vi "Write Listener Port.vi"(8 "error in (no error)":errorcluster, 10 "Listener Port":u16=6341, 11 "Server Config in":refnum<class "Server Config.lvclass">) -> (0 "error out":errorcluster, 3 "Server Config out":refnum<class "Server Config.lvclass">)   [LabVIEW 2026, in "Server Controller.lvlib" / "Server Config.lvclass"]
uses:
  Server Config.lvclass
  Server Config.lvclass/Server Config.ctl
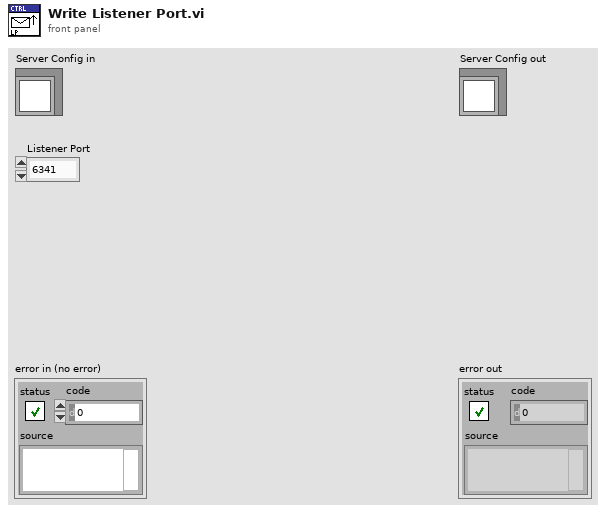
[diagram p1: front panel]
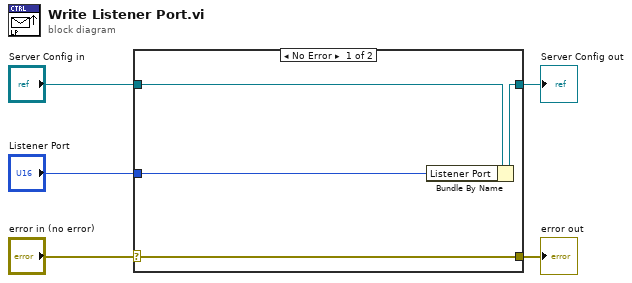
[diagram p0: block diagram]
diagram:
  n1 = case shown="No Error" "error in (no error)" {
    selector: "error in (no error)" -> [w9 w10]
    tunnel: [w9 w10] -> w4
    tunnel: [w7 w11] -> w2
    tunnel: "Server Config in" -> [w8 w11]
    tunnel: "Listener Port" -> [w6 _]
    frame No Error {
      n2 = Bundle By Name(cluster=w8, "Listener Port"=w6) -> (w7:refnum<class "Server Config.lvclass">)
    }
    frame Error {
    }
  }
  "error out" <- w4
  "Server Config out" <- w2
